vi "Data_Close.vi"(8 "Error In":errorcluster caption="错误输入", 11 "数据对象保存":refnum<file>) -> (0 "Error Out":errorcluster caption="错误输出")   [LabVIEW 2020]
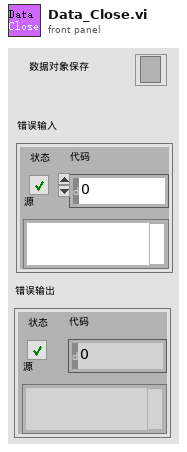
[diagram p1: front panel]
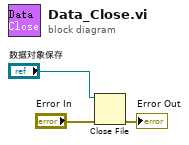
[diagram p0: block diagram]
diagram:
  n1 = Close File(refnum="数据对象保存", error in="Error In") -> (error out=→"Error Out":errorcluster)  [unwired: 1 out]
